vi "Scale Scalar DBL AO Value to I16.vi"(9 "DAC bipolar range":dbl, 11 "AO DBL value":dbl) -> (3 "AO I16 value":i16)   [LabVIEW 2020, in "Engine Simulation Toolkit System Explorer.lvlib"]
uses:
  Engine Simulation Toolkit System Explorer.lvlib
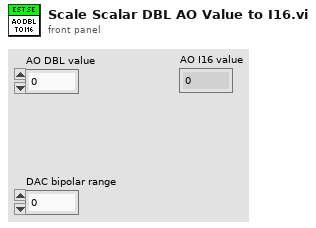
[diagram p1: front panel]
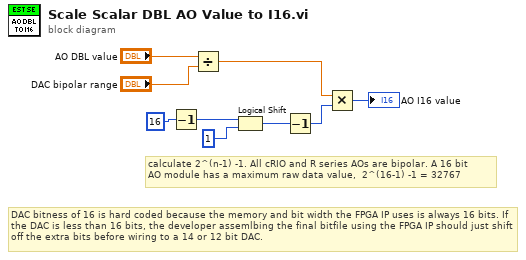
[diagram p0: block diagram]
diagram:
  # "DAC bitness of 16 is hard coded because the memory and bit width the FPGA IP uses is always 16 bits. If the DAC is less than 16 bits, the developer assemlbing the final bitfile using the FPGA IP should just shift off the extra bits before wiring to a 14 or 12 bit DAC."
  # "calculate 2^(n-1) -1. All cRIO and R series AOs are bipolar. A 16 bit\nAO module has a maximum raw data value,  2^(16-1) -1 = 32767"
  n1 = Decrement(x=u16 16 ("DAC bit resolution (16)")) -> (x-1=w7:u16)
  n2 = Divide(x="AO DBL value", y="DAC bipolar range") -> (x/y=w2:dbl)
  n3 = Logical Shift(y=w7, x=i16 1) -> (x << y=w8:i16)
  n4 = Decrement(x=w8) -> (x-1=w3:i16)
  n5 = Multiply(x=w2, y=w3) -> (x*y=→"AO I16 value":i16)
